vi "Download1 TBD file.vi"(8 "error in (no error)":errorcluster caption="错误输入（无错误）", 10 "TBC File link":string="E: \\Download TBCFIles\\E100_TS2_23_90_V3.0.tbc", 11 "VISA资源名称":refnum<visa-resource-name>="COM1") -> (0 "错误输出":errorcluster, 2 "CMD In":string[](array[string]), 3 "Result":bool)   [LabVIEW 2013]
uses:
  C:/Program Files/National Instruments/LabVIEW 2013/examples/Instrument IO/Serial/support/Serial - Settings.ctl
  <vilib>/Instr/_visa.llb/VISA Configure Serial Port (Instr).vi
panel:
  in  "路径":path
  out "读取缓冲区":string
  in  "TBC File Name 2":string="E100_TS2_23_90_V3.0.tbc"
  out "数组 2":bool[](array[boolean])
  out "添加的路径":path
  out "Feedback":string[](array[string])
  out "数组":string[](array[string])
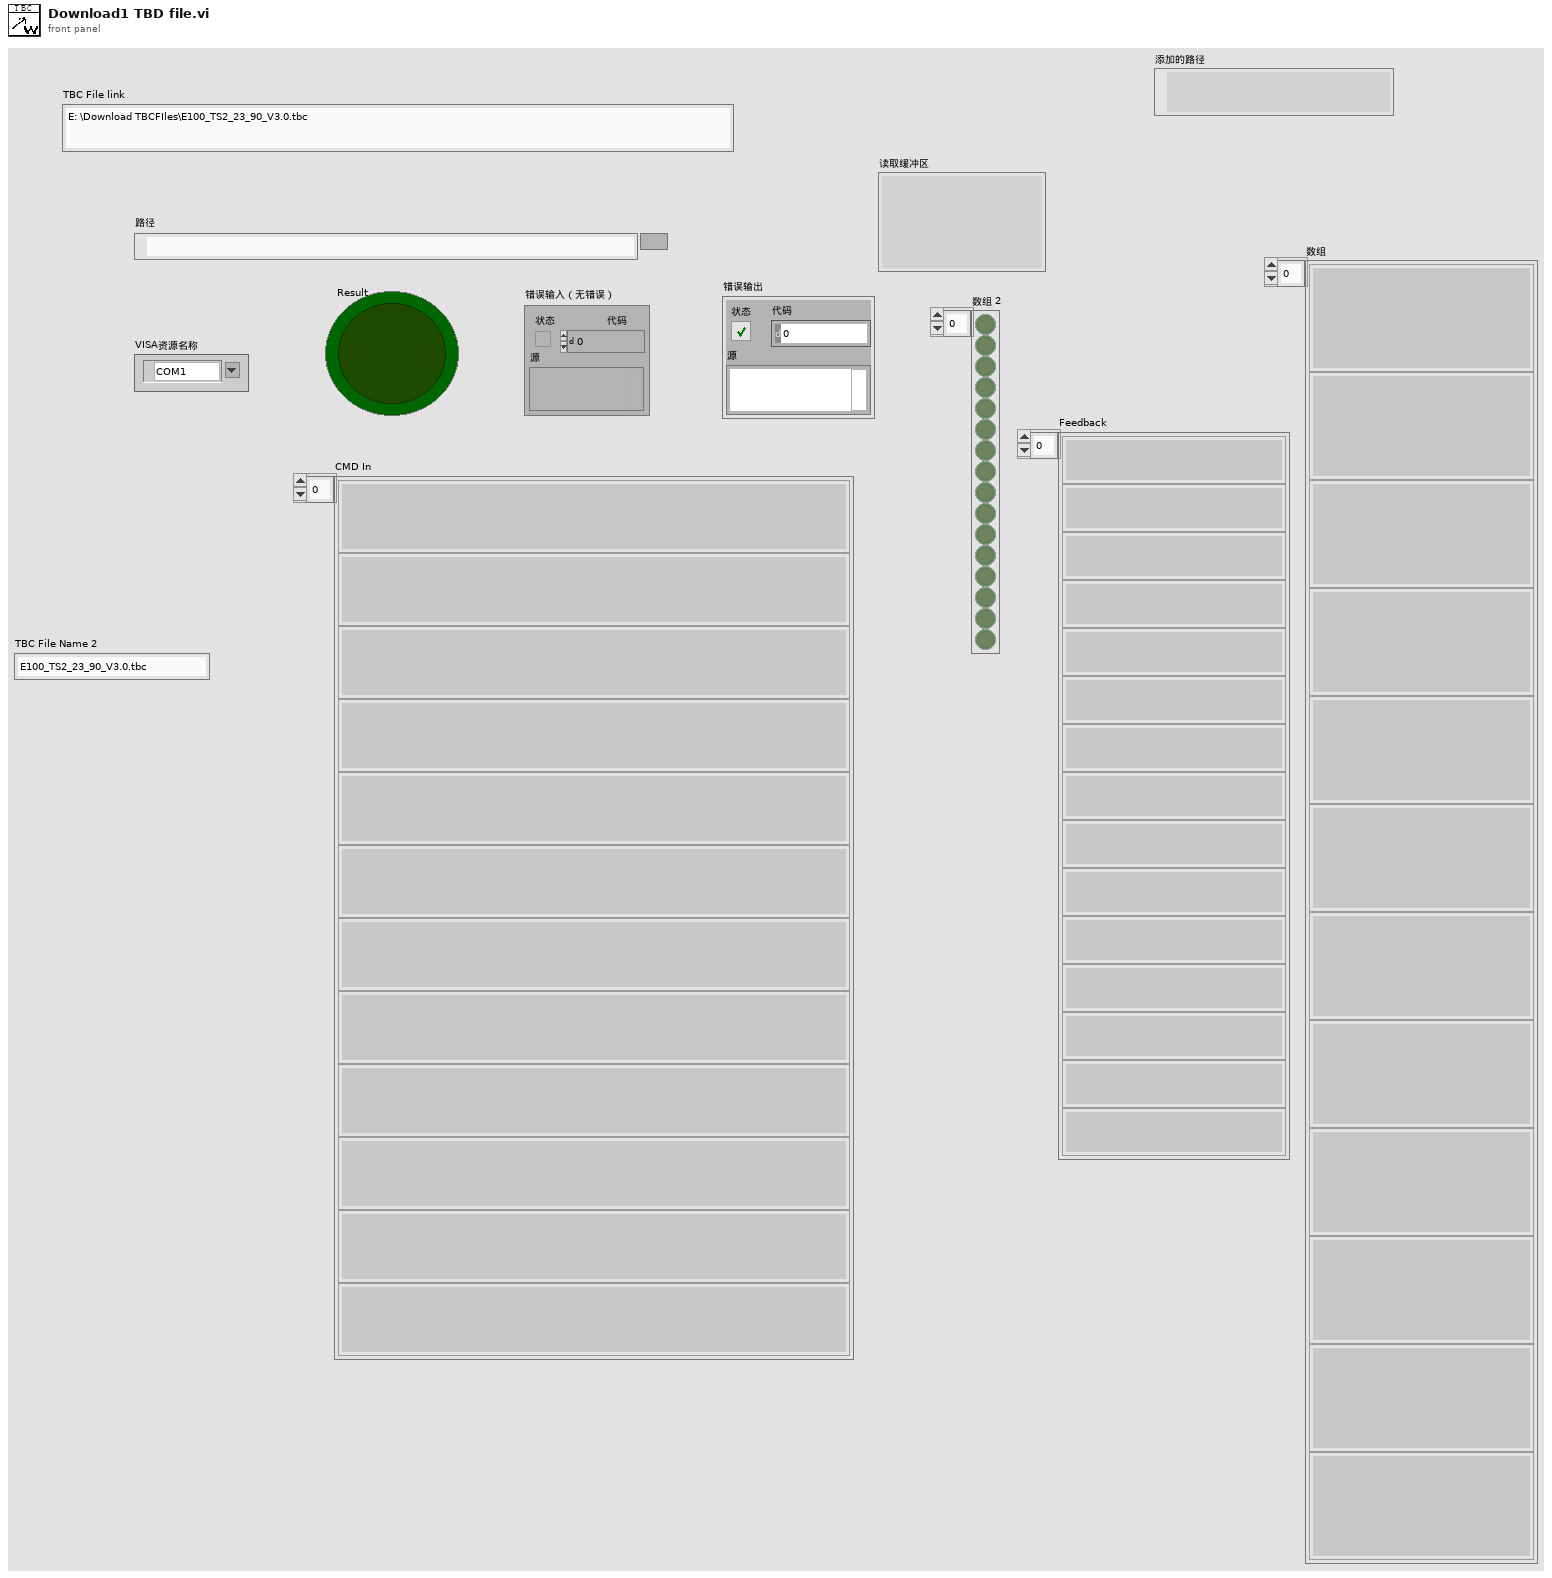
[diagram p1: front panel]
types:
  T1 = typedef "Serial - Settings.ctl" = cluster{"波特率":u32, "数据比特":u16, "奇偶":enum16{"None", "Odd", "Even", "Mark", "Space"}, "停止位":u16, "流控制":u16}
  T2 = enum32{"invalid app kind", "Development System", "Run Time System", "Student Edition", "Embedded LabVIEW", "Evaluation", "Custom"}
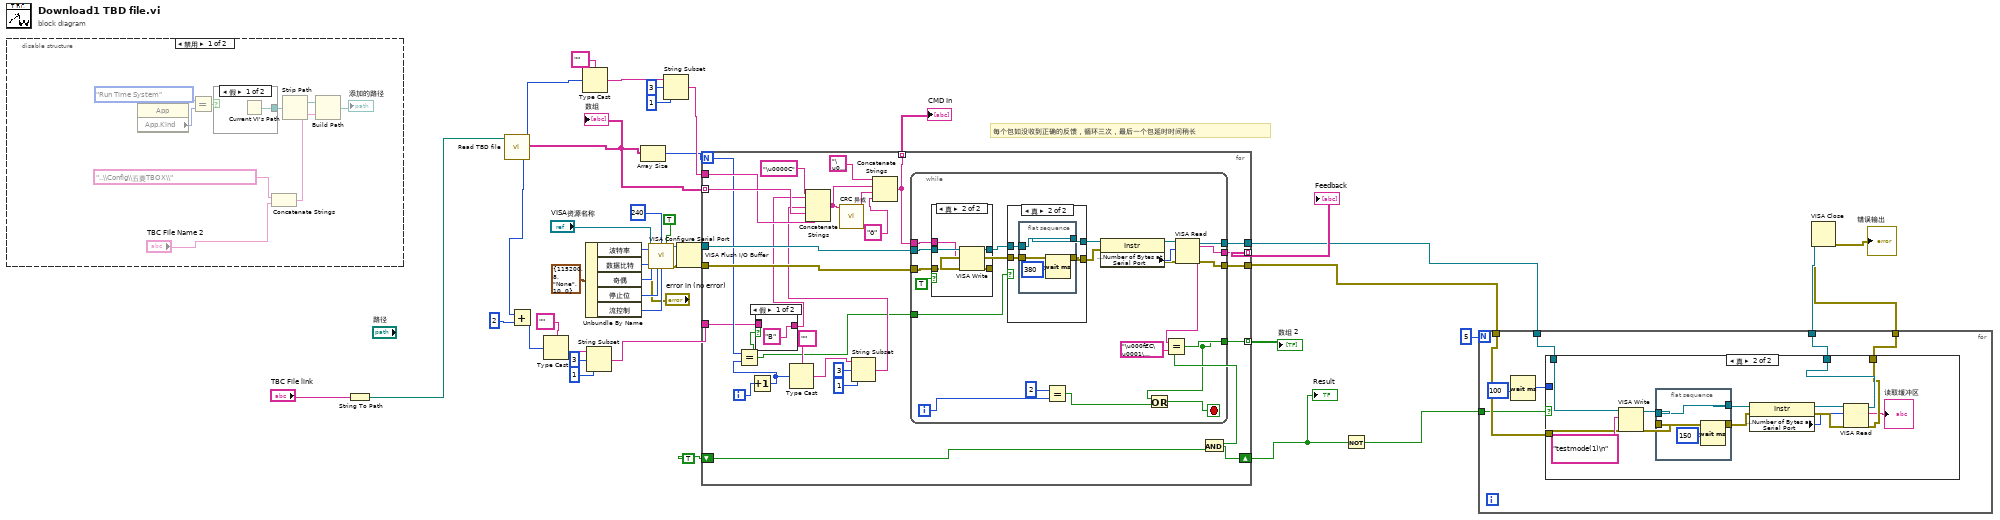
[diagram p0: block diagram]
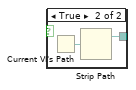
[diagram p2: hidden frame]
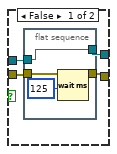
[diagram p5: hidden frame]
diagram:
  # "每个包如没收到正确的反馈，循环三次，最后一个包延时时间稍长"
  n1 = disable-structure shown="禁用" {
    frame Disabled {
      n2 = property class="App"() -> ("App.Kind"=w51:T2)  [unwired: 2 in, 2 out]
      n3 = Equal?(x=T2."Run Time System" ("y"), y=w51) -> (x = y?=w53:bool)
      n4 = case shown="假" w53 {
        tunnel: [w54 w56] -> w52
        frame False {
          n5 = Current VI's Path() -> (path=w54:path)
        }
        frame True {
          n6 = Current VI's Path() -> (path=w55:path)
          n7 = Strip Path(path=w55) -> (stripped path=w56:path)  [unwired: 1 out]
        }
      }
      n8 = Concatenate Strings("..\\Config\\五菱TBOX\\" ("连接的字符串"), "TBC File Name 2") -> (w47:string)
      n9 = Strip Path(path=w52) -> (stripped path=w49:path)  [unwired: 1 out]
      n10 = Build Path(base path=w49, name or relative path=w47) -> (appended path=→"添加的路径":path)
    }
    frame Enabled {
    }
  }
  n11 = String To Path(string="TBC File link") -> (path=w1:path)
  n12 = call "Read TBD file.vi"("文件路径（使用对话框）"=w1) -> ("末包数据量"=w14:i32, "数组"=w22:string[], "数据包数"=w28:i32)  [unwired: 7 in, 1 out]
  "数组" <- w22
  n13 = Add(x=w14, y=2 ("x-y*floor(x/y)")) -> (x+y=w15:i32)
  n14 = Type Cast(type="" ("类型"), x=w15) -> (*(type *) &x=w18:string)
  n15 = Type Cast(type="" ("类型"), x=w28) -> (*(type *) &x=w27:string)
  n16 = Unbundle By Name(T1 {"波特率"=115200, "数据比特"=8, "奇偶"=enum."None", "停止位"=10, "流控制"=0} ("串口设置")) -> ("波特率"=w40:u32, "数据比特"=w41:u16, "奇偶"=w42:enum16{"None", "Odd", "Even", "Mark", "Space"}, "停止位"=w43:u16, "流控制"=w38:u16)
  n17 = String Subset(string=w18, offset (0)=3 ("偏移量(0)"), length (rest)=1 ("长度（剩余）")) -> (substring=w16:string)
  n18 = Array Size(array=w22) -> (size(s)=w21:i32)
  n19 = call-poly "VISA Configure Serial Port"("VISA resource name"="VISA资源名称", "termination char\n(0xA = '\\n' = LF)"=u8 240 ("termination char\n(0xA = '\\n' = LF)"), "Enable Termination\nChar (T)"=TRUE ("Enable Termination\nChar (T)"), "baud rate (9600)"=w40, "data bits (8)"=w41, "parity (0:none)"=w42, "error in (no error)"="error in (no error)", "stop bits (10: 1 bit)"=w43, "flow control (0:none)"=w38) -> ("VISA resource name out"=w35:refnum<visa-resource-name>, "error out"=w36:errorcluster)  [unwired: 1 in, 4 out]
  n20 = String Subset(string=w27, offset (0)=3 ("偏移量(0)"), length (rest)=1 ("长度（剩余）")) -> (substring=w26:string)
  n21 = VISA Flush I/O Buffer(VISA resource name=w35, error in (no error)=w36) -> (VISA resource name out=w34:refnum<visa-resource-name>, error out=w33:errorcluster)  [unwired: 1 in]
  n22 = for {
    N: w21 -> [w70]
    tunnel: w34 -> [w83]
    tunnel: w33 -> [w82]
    tunnel: [w81] -> w7
    tunnel: [w80] -> w8
    tunnel: [w61] -> w31 mode=indexing
    tunnel: w22 -> [w79] mode=indexing
    tunnel: w26 -> [w76]
    tunnel: [w63] -> w23 mode=indexing
    tunnel: w16 -> [w69]
    shift-right: [w60] -> w2
    shift-left: TRUE -> [w59]
    tunnel: [w58] -> w4 mode=indexing
    i -> [w78]
    n23 = Increment(x=w78) -> (x+1=w71:i32)
    n24 = Equal?(x=w70, y=w71) -> (x = y?=w57:bool)
    n25 = case shown="假" w57 {
      tunnel: [_ w127] -> _
      tunnel: w69 -> [_ w127]
      tunnel: ["B" w127] -> w68
      frame False {
      }
      frame True {
      }
    }
    n26 = Type Cast(type="" ("类型"), x=w71) -> (*(type *) &x=w73:string)
    n27 = String Subset(string=w73, offset (0)=3 ("偏移量(0)"), length (rest)=1 ("长度（剩余）")) -> (substring=w72:string)
    n28 = Concatenate Strings("\u0000C", w68, w76, w72, w79) -> (w64:string)
    n29 = call "CRC 异或.vi"("input hex"=w64) -> ("*(类型 *) &x"=w66:string)  [unwired: 10 in]
    n30 = Concatenate Strings("\u000f" ("字符串"), w64, w66, "ð" ("字符串")) -> (w63:string)
    n31 = while {
      tunnel: w83 -> [w104]
      tunnel: w82 -> [w103]
      tunnel: [w96] -> w81
      tunnel: [w95] -> w80
      tunnel: w63 -> [w94]
      tunnel: [w93] -> w61
      tunnel: [w86] -> w58
      tunnel: w57 -> [w84]
      i -> [w90]
      stop <- w87 stop-if-true
      n32 = case shown="真" TRUE {
        tunnel: w104 -> [w120 w125]
        tunnel: [w120 w124] -> w102
        tunnel: [w119 w123] -> w100
        tunnel: w103 -> [w119 w122]
        tunnel: w94 -> [_ w121]
        frame False {
        }
        frame True {
          n33 = VISA Write(VISA resource name=w125, write buffer=w121, error in (no error)=w122) -> (VISA resource name out=w124:refnum<visa-resource-name>, error out=w123:errorcluster)  [unwired: 1 out]
        }
      }
      n34 = case shown="真" w84 {
        tunnel: w102 -> [w108 w115]
        tunnel: [w106 w114] -> w101
        tunnel: w100 -> [w107 w113]
        tunnel: [w105 w112] -> w85
        frame False {
          n35 = flat-sequence {
            tunnel: w107 -> [w111]
            tunnel: [w111] -> w105
            tunnel: w108 -> [w109]
            tunnel: [w109] -> w106
            frame #0 {
              n36 = Wait (ms)(milliseconds to wait=u32 125 ("等待时间（毫秒）")) -> ()  [unwired: 1 out]
            }
          }
        }
        frame True {
          n37 = flat-sequence {
            tunnel: w113 -> [w118]
            tunnel: [w118] -> w112
            tunnel: w115 -> [w116]
            tunnel: [w116] -> w114
            frame #0 {
              n38 = Wait (ms)(milliseconds to wait=u32 380 ("等待时间（毫秒）")) -> ()  [unwired: 1 out]
            }
          }
        }
      }
      n39 = Equal?(x=2, y=w90) -> (x = y?=w88:bool)
      n40 = property class="Instr"(reference=w101, error in=w85) -> (reference out=w97:refnum<visa-resource-name>, error out=w98:errorcluster, "Serial Settings:Number of Bytes at Serial Port"=w99:u32)
      n41 = VISA Read(VISA resource name=w97, byte count=w99, error in (no error)=w98) -> (VISA resource name out=w95:refnum<visa-resource-name>, read buffer=w93:string, error out=w96:errorcluster)  [unwired: 1 out]
      n42 = Equal?(x=w93, y="\u000f€C\u0001\u0001Âð") -> (x = y?=w86:bool)
      n43 = Or(x=w86, y=w88) -> (x .or. y?=w87:bool)
    }
    n44 = And(x=w58, y=w59) -> (x .and. y?=w60:bool)
  }
  "Feedback" <- w31
  "CMD In" <- w23
  "Result" <- w2
  "数组 2" <- w4
  n45 = Not(x=w2) -> (.not. x?=w3:bool)
  n46 = for {
    N: 5 -> [_]
    tunnel: w8 -> [w134]
    tunnel: w7 -> [w133]
    tunnel: [w132] -> w6
    tunnel: [w131] -> w5
    tunnel: w3 -> [w129]
    n47 = Wait (ms)(milliseconds to wait=u32 100 ("等待时间（毫秒）")) -> (millisecond timer value=w128:u32)
    n48 = case shown="真" w129 {
      tunnel: w134 -> [w136 w149]
      tunnel: w133 -> [w135 w147]
      tunnel: [w136 w139] -> w132
      tunnel: [w135 w138] -> w131
      tunnel: w128 -> [_ _]
      frame False {
      }
      frame True {
        n49 = VISA Write(VISA resource name=w149, write buffer="testmode(1)\n" ("写入缓冲区"), error in (no error)=w147) -> (VISA resource name out=w141:refnum<visa-resource-name>, error out=w140:errorcluster)  [unwired: 1 out]
        n50 = flat-sequence {
          tunnel: w140 -> [w152]
          tunnel: [w152] -> w143
          tunnel: w141 -> [w150]
          tunnel: [w150] -> w142
          frame #0 {
            n51 = Wait (ms)(milliseconds to wait=u32 150 ("等待时间（毫秒）")) -> ()  [unwired: 1 out]
          }
        }
        n52 = property class="Instr"(reference=w142, error in=w143) -> (reference out=w146:refnum<visa-resource-name>, error out=w145:errorcluster, "Serial Settings:Number of Bytes at Serial Port"=w144:u32)
        n53 = VISA Read(VISA resource name=w146, byte count=w144, error in (no error)=w145) -> (VISA resource name out=w139:refnum<visa-resource-name>, read buffer=→"读取缓冲区":string, error out=w138:errorcluster)  [unwired: 1 out]
      }
    }
  }
  n54 = VISA Close(VISA resource name=w6, error in (no error)=w5) -> (error out=→"错误输出":errorcluster)
